vi "Write Server RPC Methods.vi"(8 "error in (no error)":errorcluster, 10 "Server RPC Methods":T1, 11 "SignalGeneratorService in":refnum<class "BLSClimateChamberTemplateService.lvclass">) -> (0 "error out":errorcluster, 3 "SignalGeneratorService out":refnum<class "BLSClimateChamberTemplateService.lvclass">)   [LabVIEW 2023, in "BLSClimateChamberTemplateService_server.lvlib" / "BLSClimateChamberTemplateService.lvclass"]
uses:
  BLSClimateChamberTemplateService.lvclass
  typeDefs/Server gRPC UEs.ctl
  <vilib>/gRPC/LabVIEW gRPC Library/Server API/typeDefs/gRPCId Cluster.ctl
  <vilib>/gRPC/LabVIEW gRPC Library/Shared/grpcId.ctl
  BLSClimateChamberTemplateService.lvclass/BLSClimateChamberTemplateService.ctl
  <vilib>/gRPC/LabVIEW gRPC Library/grpc-lvsupport-release.lvlib
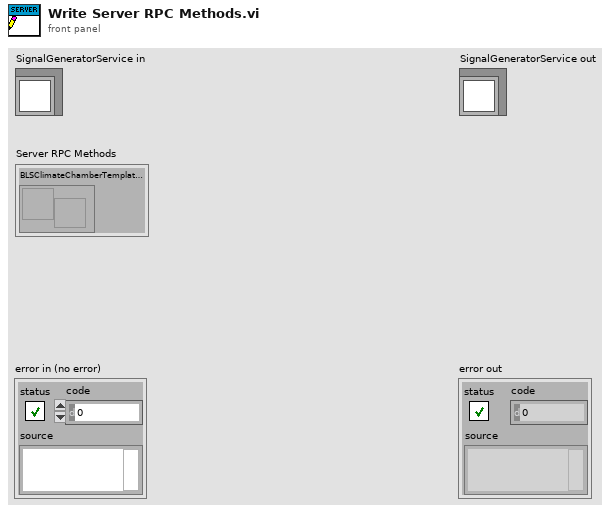
[diagram p1: front panel]
types:
  T1 = typedef "BLSClimateChamberTemplateService_server.lvlib/BLSClimateChamberTemplateService.lvclass/Server gRPC UEs.ctl" = cluster{"BLSClimateChamberTemplateService SetNumber gRPC UE":refnum<user-event>}
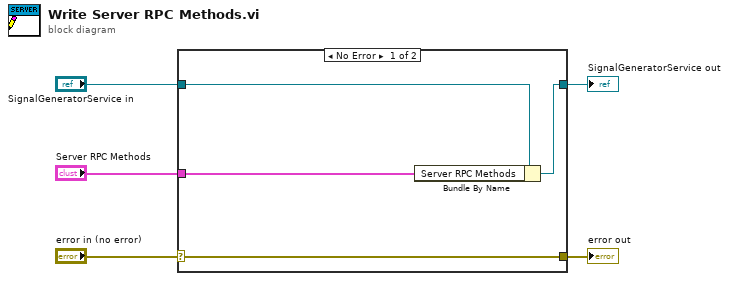
[diagram p0: block diagram]
diagram:
  n1 = case shown="No Error" "error in (no error)" {
    selector: "error in (no error)" -> [w9 w10]
    tunnel: [w9 w10] -> w4
    tunnel: [w7 w11] -> w2
    tunnel: "SignalGeneratorService in" -> [w8 w11]
    tunnel: "Server RPC Methods" -> [w6 _]
    frame No Error {
      n2 = Bundle By Name(cluster=w8, "Server RPC Methods"=w6) -> (w7:refnum<class "BLSClimateChamberTemplateService.lvclass">)
    }
    frame Error {
    }
  }
  "error out" <- w4
  "SignalGeneratorService out" <- w2
